vi "Register VI(s).vi"   [LabVIEW 2017, in "JKI Simple Localization.lvlib"]
doc: "Register VI(s) to the localizer's registry. Automatically applies the current language to these VIs."
uses:
  JKI Simple Localization.lvlib
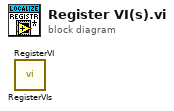
[diagram p0: block diagram]
diagram:
  n1 = call "RegisterVIs.vi"() -> ()  [unwired: 10 in, 2 out]
  n2 = call "RegisterVI.vi"() -> ()  [unwired: 10 in, 2 out]
